vi "Factory.vi"(0 "Obj in":refnum<class "AM.lvclass">, 7 "Variant":variant, 9 "Prefix":string, 11 "error in (no error)":errorcluster) -> (4 "Obj out":refnum<class "AM.lvclass">, 8 "Type":string, 15 "error out":errorcluster)   [LabVIEW 2020, in "AM.lvclass"]
uses:
  AM.lvclass
  Koop/KObject Class/KObject.lvclass
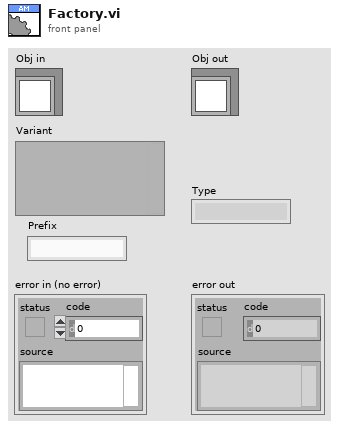
[diagram p1: front panel]
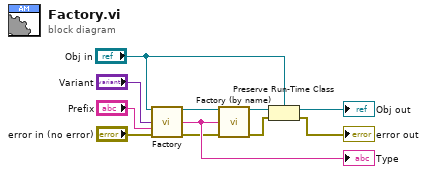
[diagram p0: block diagram]
diagram:
  n1 = call-parent "Factory.vi"("KObject in"="Obj in", "Variant"="Variant", "Prefix"="Prefix", "error in (no error)"="error in (no error)") -> ("KObject out"=w8:refnum<class "AM.lvclass">, "Type"=w7:string, "error out"=w6:errorcluster)  [unwired: 9 in]
  "Type" <- w7
  n2 = call "Factory (by name).vi"("Obj in"=w8, "Class Name"=w7, "error in (no error)"=w6) -> ("Obj out"=w4:refnum<class "AM.lvclass">, "error out"=w5:errorcluster)  [unwired: 11 in]
  n3 = Preserve Run-Time Class(object in=w4, error in=w5, 2:"Obj in") -> (object out=→"Obj out":refnum<class "AM.lvclass">, error out=→"error out":errorcluster)
